vi "ShowWizard.vi"(3 "String":string, 4 "error in (no error)":errorcluster, 5 "hWnd":u32) -> (2 "error out":errorcluster)   [LabVIEW 2009]
doc: "Show the DAQNavi Wizard. User can select scenario, select device and config."
uses:
  BioLvWizard.dll
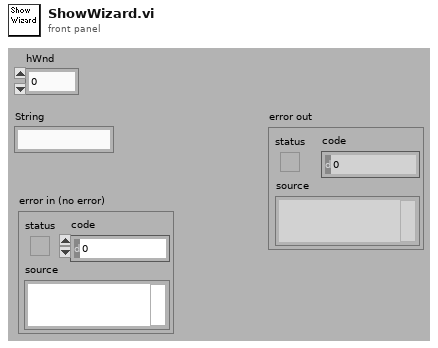
[diagram p1: front panel]
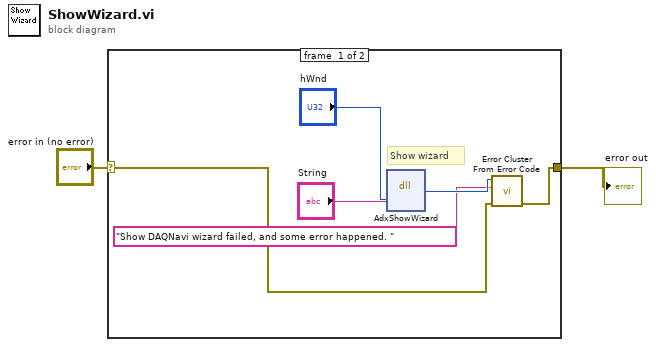
[diagram p0: block diagram]
diagram:
  n1 = case shown="No Error" "error in (no error)" {
    selector: "error in (no error)" -> [w5 w9]
    tunnel: [w3 w9] -> w1
    frame #0 {
      # "Show wizard"
      n2 = dll-call lib="BioLvWizard.dll" fn="AdxShowWizard"("host_wnd"="hWnd", "cfg_file_path"="String") -> ("return type"=w6:i32)  [unwired: 5 in, 2 out]
      n3 = call <vilib>:"Error Cluster From Error Code.vi"("error in (no error)"=w5, "error message (\"\")"="Show DAQNavi wizard failed, and some error happened. " ("error message (\"\")"), "error code (0)"=w6) -> ("error out"=w3:errorcluster)  [unwired: 1 in, 5 out]
    }
    frame #1 {
    }
  }
  "error out" <- w1
